vi "HSMS Request And Wait For Reply.vi"(8 "error in (no error)":errorcluster, 10 "SECS-II Class In":refnum<class "SECS-II Class.lvclass">, 11 "HSMS Class in":refnum<class "HSMS Class.lvclass">) -> (0 "error out":errorcluster, 1 "Timeout?":bool, 2 "SECS-II Class Out":refnum<class "SECS-II Class.lvclass">, 3 "HSMS Class out":refnum<class "HSMS Class.lvclass">)   [LabVIEW 2020, in "SECS Communication.lvlib" / "HSMS Class.lvclass"]
uses:
  HSMS Class.lvclass
  SECS-II Class/SECS-II Class.lvclass
  Command Data.ctl
  HSMS Class.lvclass/HSMS Class.ctl
  SECS-II Class/SECS-II Class.lvclass/SECS-II Class.ctl
  SECS-II Class/Read Function.vi
  Read T3(Reply Timeout).vi
  SECS-II Class/Write System Btyes.vi
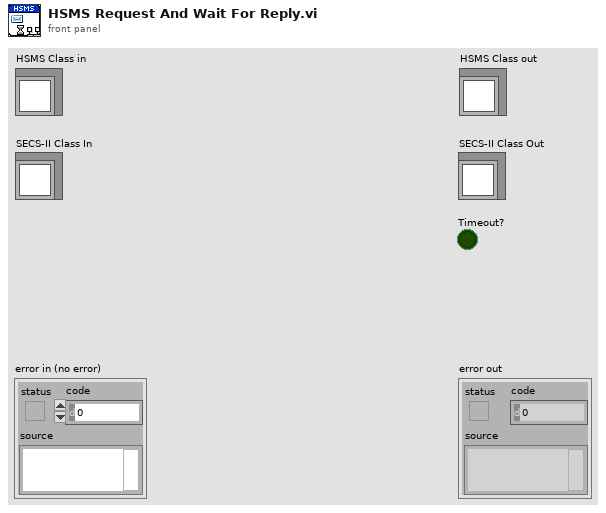
[diagram p1: front panel]
types:
  T1 = typedef "SECS Communication.lvlib/HSMS Class.lvclass/Command Data.ctl" = cluster{"SECS-II Class":refnum<class "SECS-II Class.lvclass">, "Reply Notifier":refnum<notifier>}
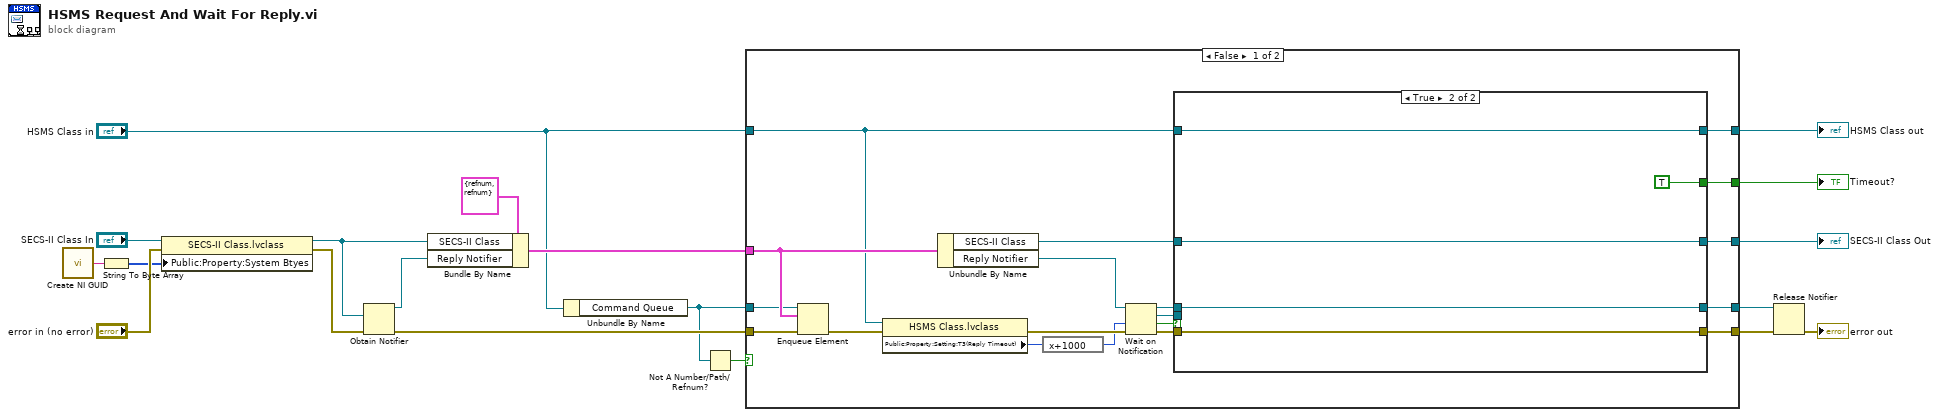
[diagram p0: block diagram]
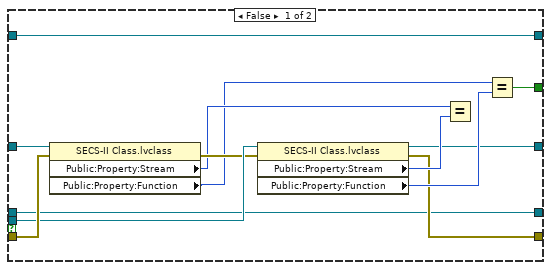
[diagram p2: hidden frame]
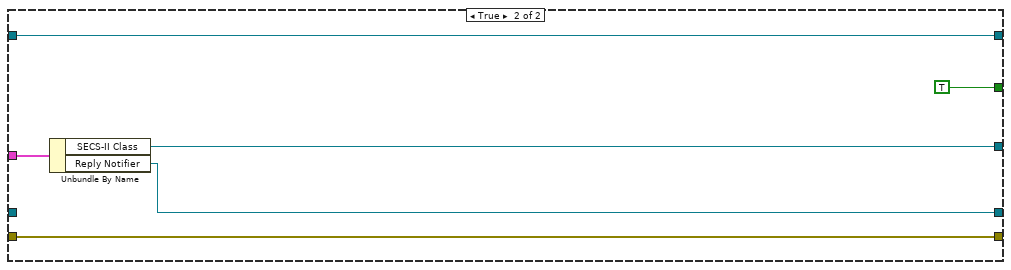
[diagram p3: hidden frame]
diagram:
  n1 = call <vilib>:"Create NI GUID.vi"() -> ("NI GUID"=w10:string)
  n2 = String To Byte Array(string=w10) -> (unsigned byte array=w9:u8[])
  n3 = property class="SECS-II Class.lvclass"(reference="SECS-II Class In", error in="error in (no error)", "Public:Property:System Btyes"=w9) -> (reference out=w11:refnum<class "SECS-II Class.lvclass">, error out=w12:errorcluster)
  n4 = Obtain Notifier(notification data type=w11, error in (no error)=w12) -> (notifier out=w18:refnum<notifier>, error out=w17:errorcluster)  [unwired: 2 in, 1 out]
  n5 = Bundle By Name(cluster=T1 {"SECS-II Class"=refnum, "Reply Notifier"=refnum} ("element"), "SECS-II Class"=w11, "Reply Notifier"=w18) -> (w16:T1)
  n6 = Unbundle By Name("HSMS Class in") -> ("Command Queue"=w2:refnum<queue>)
  n7 = Not A Number/Path/Refnum?(number/path/refnum=w2) -> (NaN/Path/Refnum?=w1:bool)
  n8 = case shown="False" w1 {
    tunnel: w17 -> [w38 w62]
    tunnel: w16 -> [w37 w61]
    tunnel: "HSMS Class in" -> [w27 w60]
    tunnel: [w26 w60] -> w7
    tunnel: [w24 w57] -> w6
    tunnel: [w23 w62] -> w5
    tunnel: [w22 w58] -> w4
    tunnel: [w21 TRUE] -> w3
    tunnel: w2 -> [w20 _]
    frame False {
      n9 = Enqueue Element(queue=w20, element=w37, error in (no error)=w38) -> (error out=w36:errorcluster)  [unwired: 1 in, 2 out]
      n10 = property class="HSMS Class.lvclass"(reference=w27, error in=w36) -> (error out=w35:errorcluster, "Public:Property:Setting:T3(Reply Timeout)"=w34:i32)  [unwired: 1 out]
      n11 = Unbundle By Name(w37) -> ("SECS-II Class"=w29:refnum<class "SECS-II Class.lvclass">, "Reply Notifier"=w32:refnum<notifier>)
      n12 = expression code="x+1000"(w34) -> (w33:i32)
      n13 = Wait on Notification(notifier=w32, timeout in ms (-1)=w33, error in (no error)=w35) -> (notifier out=w25:refnum<notifier>, notification=w30:refnum<class "SECS-II Class.lvclass">, timed out?=w28:bool, error out=w31:errorcluster)  [unwired: 1 in]
      n14 = case shown="True" w28 {
        tunnel: w31 -> [w51 w54]
        tunnel: w30 -> [w49 _]
        tunnel: w29 -> [w50 w55]
        tunnel: w27 -> [w45 w56]
        tunnel: [w45 w56] -> w26
        tunnel: w25 -> [w42 w53]
        tunnel: [w42 w53] -> w24
        tunnel: [w41 w55] -> w22
        tunnel: [w43 w54] -> w23
        tunnel: [w39 TRUE] -> w21
        frame False {
          n15 = property class="SECS-II Class.lvclass"(reference=w50, error in=w51) -> (error out=w48:errorcluster, "Public:Property:Stream"=w46:u8, "Public:Property:Function"=w40:u8)  [unwired: 1 out]
          n16 = property class="SECS-II Class.lvclass"(reference=w49, error in=w48) -> (reference out=w41:refnum<class "SECS-II Class.lvclass">, error out=w43:errorcluster, "Public:Property:Stream"=w47:u8, "Public:Property:Function"=w44:u8)
          n17 = Equal?(x=w46, y=w47) -> ()  [unwired: 1 out]
          n18 = Equal?(x=w40, y=w44) -> (x = y?=w39:bool)
        }
        frame True {
        }
      }
    }
    frame True {
      n19 = Unbundle By Name(w61) -> ("SECS-II Class"=w58:refnum<class "SECS-II Class.lvclass">, "Reply Notifier"=w57:refnum<notifier>)
    }
  }
  "HSMS Class out" <- w7
  "SECS-II Class Out" <- w4
  "Timeout?" <- w3
  n20 = Release Notifier(notifier=w6, error in (no error)=w5) -> (error out=→"error out":errorcluster)  [unwired: 1 in, 2 out]
